vi "raven_decoder.vi"(0 "Array (Time vs Pad) In":u16[][](array[numeric]), 1 "Packeges Array":u16[](array[numeric]), 2 "Timestamp number":i32, 3 "Digital 1 threshold":i32) -> (7 "Array (Time vs Pad) Out":u16[][](array[numeric]))   [LabVIEW 2013]
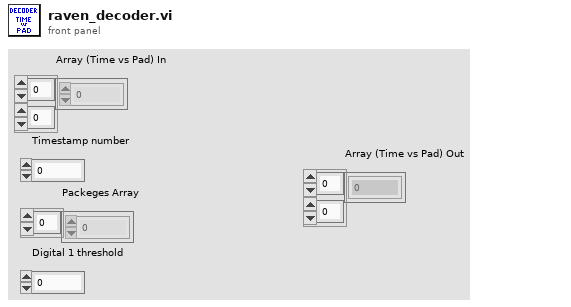
[diagram p1: front panel]
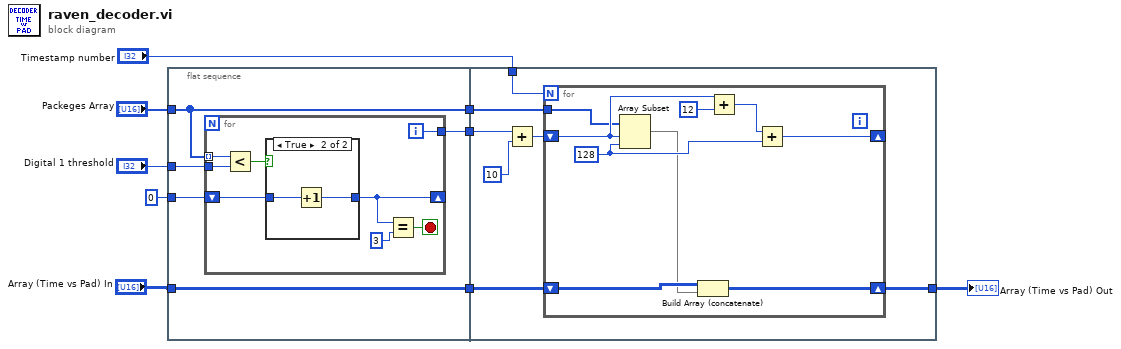
[diagram p0: block diagram]
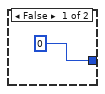
[diagram p2: hidden frame]
diagram:
  n1 = flat-sequence {
    tunnel: "Packeges Array" -> [w11]
    tunnel: "Digital 1 threshold" -> [w14]
    tunnel: [w11] -> w9
    tunnel: [w13] -> w8
    tunnel: 0 ("Numeric") -> [w12]
    tunnel: "Array (Time vs Pad) In" -> [w10]
    tunnel: [w10] -> w2
    tunnel: w9 -> [w28]
    tunnel: w8 -> [w30]
    tunnel: "Timestamp number" -> [w32]
    tunnel: [w27] -> w3
    tunnel: w2 -> [w26]
    frame #0 {
      n2 = for {
        tunnel: w11 -> [w21] mode=indexing
        tunnel: w14 -> [w20]
        shift-right: [w16] -> _
        shift-left: w12 -> [w19]
        tunnel: [w17] -> w13
        i -> [w17]
        stop <- w18 stop-if-true
        n3 = Less?(x=w21, y=w20) -> (x < y?=w22:bool)
        n4 = case shown="True" w22 {
          tunnel: w19 -> [_ w25]
          tunnel: [0 w24] -> w16
          frame False {
          }
          frame True {
            n5 = Increment(x=w25) -> (x+1=w24:i32)
          }
        }
        n6 = Equal?(x=w16, y=3 ("x")) -> (x = y?=w18:bool)
      }
    }
    frame #1 {
      n7 = Add(x=w30, y=10) -> (x+y=w29:i32)
      n8 = for {
        N: w32 -> [_]
        tunnel: w28 -> [w37]
        shift-right: [w41] -> _
        shift-left: w29 -> [w38]
        shift-right: [w36] -> w27
        shift-left: w26 -> [w35]
        w34 = 128 ("length")
        n9 = Array Subset(array=w37, index=w38, length=w34) -> (w33:u16[])
        n10 = Build Array (concatenate)(w35, w33) -> (w36:u16[][])
        n11 = Add(x=w38, y=12) -> (x+y=w39:i32)
        n12 = Add(x=w39, y=w34) -> (x+y=w41:i32)
      }
    }
  }
  "Array (Time vs Pad) Out" <- w3
